vi "Save Waveform Memory.vi"(8 "error in (no error)":errorcluster, 9 "Waveform Memory (9: Memory 1)":u16(ring)=9 items=["Memory 1"=9, "Memory 2"=10, "Memory 3"=11, "Memory 4"=12], 10 "Measurement Source (1: Channel 1)":u16(ring)=1 items=["Channel 1"=1, "Channel 2"=2, "Channel 3"=3, "Channel 4"=4, "Function 1"=5, "Function 2"=6, "Function 3"=7, "Function 4"=8, "Memory 1"=9, "Memory 2"=10, "Memory 3"=11, "Memory 4"=12, "Differential 1"=61, "Differential 2"=62, "Common 1"=71, "Common 2"=72, "Clock"=15, "MTrend"=16, "MSpectrum"=17], 11 "VISA resource name":refnum<visa-resource-name>) -> (0 "error out":errorcluster, 3 "VISA resource name out":refnum<visa-resource-name>)   [LabVIEW 2020, in "Agilent 90000 Series.lvlib"]
doc: "Stores the specified channel, waveform memory, or function to the waveform memory. The channel or function must be enabled or an error status is returned. User can save waveform to waveform memories whether the waveform memory is displayed or not."
uses:
  Agilent 90000 Series.lvlib
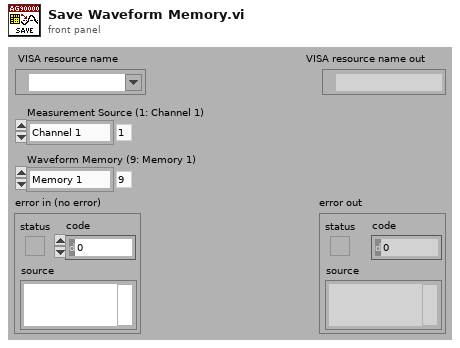
[diagram p1: front panel]
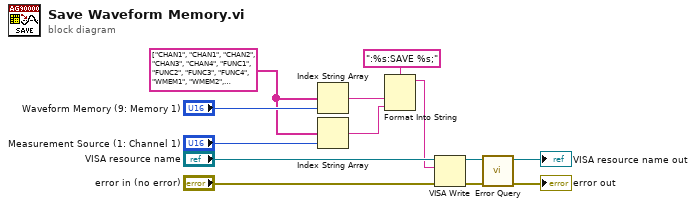
[diagram p0: block diagram]
diagram:
  w1 = string[] ["CHAN1", "CHAN1", "CHAN2", "CHAN3", "CHAN4", "FUNC1", "FUNC2", "FUNC3", "FUNC4", "WMEM1", "WMEM2", "WMEM3", "WMEM4", "AUX", "LINE", "CLOC", "MTR", "MSP", "EQU", "NONE", "DIG0", "DIG1", "DIG2", "DIG3", "DIG4", "DIG5", "DIG6", "DIG7", "DIG8", "DIG9", "DIG10", "DIG11", "DIG12", "DIG13", "DIG14", "DIG15", "", "", "", "", "", "POD1", "POD2", "", "", "", "", "", "", "", "", "BUS1", "BUS2", "BUS3", "BUS4", "", "", "", "", "", "", "DIFF1", "DIFF2", "", "", "", "", "", "", "", "", "COMM3", "COMM4"]
  n1 = Index String Array(1:"Waveform Memory (9: Memory 1)", 2:w1) -> (0:w3:string)  [unwired: 1 out]
  n2 = Index String Array(1:"Measurement Source (1: Channel 1)", 2:w1) -> (0:w4:string)  [unwired: 1 out]
  n3 = Format Into String(format string=":%s:SAVE %s;", w3, w4) -> (resulting string=w2:string)  [unwired: 2 in, 1 out]
  n4 = VISA Write(VISA resource name="VISA resource name", write buffer=w2, error in (no error)="error in (no error)") -> (VISA resource name out=w9:refnum<visa-resource-name>, error out=w8:errorcluster)  [unwired: 1 out]
  n5 = call "Error Query.vi"("error in (no error)"=w8, "VISA resource name"=w9) -> ("error out"=→"error out":errorcluster, "VISA resource name out"=→"VISA resource name out":refnum<visa-resource-name>)  [unwired: 8 out]
